vi "Get INI Section.vi"(4 "section name":string="desktop", 5 "file content":string="[windows]\nspooler=no\nNetWarn=1\nNetMessage=Yes\nload=c:\\windows\\number9\\hawkeye.exe C:\\MOUSE\\pointer.exe\n\nrun=c:\\DELL\\WINBATCH.EXE\nBeep=yes\nNullPort=None\ndevice=\nBorderWidth=3\nCursorBlinkRate=530\nDoubleClickSpeed=452\nPrograms=com exe bat pif\nDocuments=\nDeviceNotSelectedTimeout=15\nTransmissionRetryTimeout=45\nKeyboardDelay=2\nKeyboardSpeed=31\nScreenSaveActive=0\nScreenSaveTimeOut=120\n\n[Desktop]\noldwallpaper=dell1.bmp\nPattern=(None)\nTileWallpaper=1\nGridGranularity=0\n\n[Extensions]\ncal=calendar.exe ^.cal\ncrd=cardfile.exe ^.crd\ntrm=terminal.exe ^.trm\ntxt=notepad.exe ^.txt\nini=notepad.exe ^.ini\npcx=pbrush.exe ^.pcx\nbmp=pbrush.exe ^.bmp\nwri=write.exe ^.wri\nrec=recorder.exe ^.rec\nhlp=winhelp.exe ^.hlp\n\n[intl]\nsLanguage=enu\nsCountry=United States\niCountry=1\niDate=0\niTime=0\niTLZero=0\niCurrency=0\niCurrDigits=2\niNegCurr=0\niLzero=1\niDigits=2\niMeasure=1\ns1159=AM\ns2359=PM\nsCurrency=$\nsThousand=,\nsDecimal=.\nsDate=/\nsTime=:\nsList=,\nsShortDate=M/d/yy\nsLongDate=dddd, MMMM dd, yyyy\n\n[ports]\n; A line with [filename].PRN followed by an equal sign causes\n; [filename] to appear in the Control Panel's Printer Configuration dialog\n; box. A printer connected to [filename] directs its output into this file.\nLPT1:=\nLPT2:=\nLPT3:=\nCOM1:=9600,n,8,1,x\nCOM2:=9600,n,8,1,x\nCOM3:=9600,n,8,1,x\nCOM4:=9600,n,8,1,x\nEPT:=\nFILE:=\nLPT1.DOS=\nLPT2.DOS=\n\n[FontSubstitutes]\nHelv=MS Sans Serif\nTms Rmn=MS Serif\nTimes=Times New Roman\nHelvetica=Arial\n\n[TrueType]\n\n[Sounds]\nRingOut=ringout.wav,Chat Outgoing Ring\nRingIn=ringin.wav,Chat Incoming Ring\nSystemDefault=ding.wav, Default Beep\nSystemExclamation=chord.wav, Exclamation\nSystemStart=tada.wav, Windows Start\nSystemExit=chimes.wav, Windows Exit\nSystemHand=chord.wav, Critical Stop\nSystemQuestion=chord.wav, Question\nSystemAsterisk=chord.wav, Asterisk\n\n[mci extensions]\nwav=waveaudio\nmid=sequencer\nrmi=sequencer\n\n[Compatibility]\nTURBOTAX=0x00080000\nW4GLR=0x4000\nW4GL=0x4000\nNETSET2=0x0100\nGUIDE=0x1000\nEXCEL=0x1000\nAPORIA=0x0100\nED=0x00010000\nPLUS=0x1000\nPR2=0x2000\nCHARISMA=0x2000\nWINSIM=0x2000\nDRAW=0x2000\nPLANNER=0x2000\nDESIGNER=0x2000\nPM4=0x2000\nMILESV3=0x1000\n_BNOTES=0x24000\nMCOURIER=0x0800\nVISION=0x0040\nPACKRAT=0x0800\nWIN2WRS=0x1210\nVB=0x0200\nTME=0x0100\nJW=0x42080\nCP=0x0040\nPIXIE=0x0040\nREM=0x8022\nAMIPRO=0x0010\nCCMAIL=0x0008\nWPWINFIL=0x0006\nNOTSHELL=0x0001\n\n[Microsoft Word 2.0]\nHPDSKJET=+1\n\n[wt4gpi8s56bz]\nArial (TrueType)=ARIAL.FOT\nArial Bold (TrueType)=ARIALBD.FOT\nArial Bold Italic (TrueType)=ARIALBI.FOT\nArial Italic (TrueType)=ARIALI.FOT\nCourier New (TrueType)=COUR.FOT\nCourier New Bold (TrueType)=COURBD.FOT\nCourier New Bold Italic (TrueType)=COURBI.FOT\nCourier New Italic (TrueType)=COURI.FOT\nTimes New Roman (TrueType)=TIMES.FOT\nTimes New Roman Bold (TrueType)=TIMESBD.FOT\nTimes New Roman Bold Italic (TrueType)=TIMESBI.FOT\nTimes New Roman Italic (TrueType)=TIMESI.FOT\nWingDings (TrueType)=WINGDING.FOT\nMS Sans Serif 8,10,12,14,18,24 (VGA res)=SSERIFE.fon\nCourier 10,12,15 (VGA res)=COURE.fon\nMS Serif 8,10,12,14,18,24 (VGA res)=SERIFE.fon\nSymbol 8,10,12,14,18,24 (VGA res)=SYMBOLE.fon\nRoman (Plotter)=ROMAN.FON\nScript (Plotter)=SCRIPT.FON\nModern (Plotter)=MODERN.FON\nSmall Fonts (VGA res)=SMALLE.fon\nHelv 8,10,12,14,18,24 (1280 res)=HELVF.FON\nTms Rmn 8,10,12,14,18,24 (1280 res)=TMSRF.FON\nCourier 10,12,15 (1280 res)=COURF.FON\nSymbol (TrueType)=SYMBOL.FOT\n\n[embedding]\nSoundRec=Sound,Sound,SoundRec.exe,picture\nPackage=Package,Package,packager.exe,picture\nPBrush=Paintbrush Picture,Paintbrush Picture,pbrush.exe,picture\n\n[winsetup]\nsource_disk_path=a:\\\n") -> (0 "after section":string, 1 "section":string[](array[string]), 2 "before section":string)   [LabVIEW 2020, in "NI_FTP.lvlib"]
uses:
  <vilib>/FTP/NI_FTP.lvlib
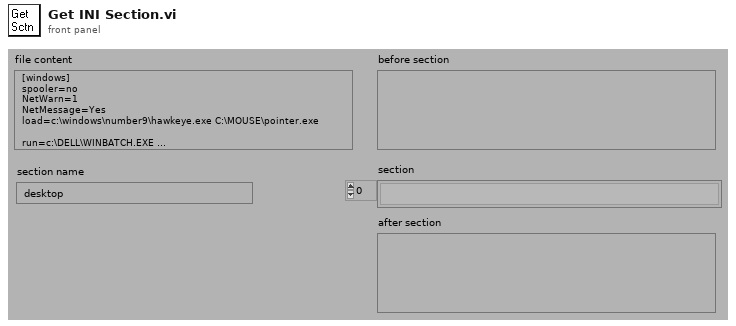
[diagram p1: front panel]
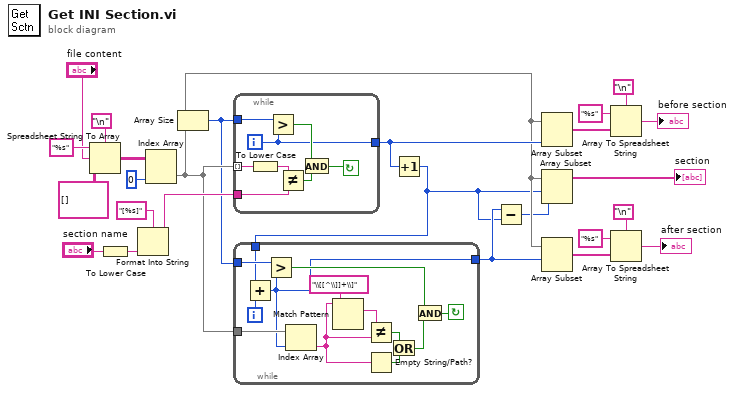
[diagram p0: block diagram]
diagram:
  n1 = Spreadsheet String To Array(delimiter (Tab)="\n", format string="%s", spreadsheet string="file content", array type (2D Dbl)=string[][] []) -> (array=w22:string[][])
  n2 = To Lower Case(string="section name") -> (all lower case string=w18:string)
  n3 = Format Into String(format string="[%s]", w18) -> (resulting string=w16:string)  [unwired: 2 in, 1 out]
  n4 = Index Array(array=w22, index (col)=0) -> (element=w6:string[])  [unwired: 1 in]
  n5 = Array Size(array=w6) -> (size(s)=w3:i32)
  n6 = while {
    tunnel: [w26] -> w15
    tunnel: w3 -> [w30]
    tunnel: w16 -> [w32]
    tunnel: w6 -> [w33] mode=indexing
    i -> [w26]
    stop <- w27 continue-if-true
    n7 = To Lower Case(string=w33) -> (all lower case string=w31:string)
    n8 = Greater?(x=w30, y=w26) -> (0:w29:bool)
    n9 = Not Equal?(x=w31, y=w32) -> (x != y?=w28:bool)
    n10 = And(x=w29, y=w28) -> (x .and. y?=w27:bool)
  }
  n11 = Increment(x=w15) -> (x+1=w1:i32)
  n12 = while {
    tunnel: [w34] -> w2
    tunnel: w1 -> [w36]
    tunnel: w3 -> [w44]
    tunnel: w6 -> [w43]
    i -> [w45]
    stop <- w40 continue-if-true
    n13 = Add(x=w36, y=w45) -> (x+y=w34:i32)
    n14 = Greater?(x=w44, y=w34) -> (0:w41:bool)
    n15 = Index Array(array=w43, index=w34) -> (element=w39:string)
    n16 = Match Pattern(string=w39, regular expression="\\[[^\\]]+\\]") -> (match substring=w42:string)  [unwired: 4 out]
    n17 = Not Equal?(x=w42, y=w39) -> (x != y?=w37:bool)
    n18 = Empty String/Path?(string/path=w39) -> (empty?=w35:bool)
    n19 = Or(x=w37, y=w35) -> (x .or. y?=w38:bool)
    n20 = And(x=w41, y=w38) -> (x .and. y?=w40:bool)
  }
  n21 = Subtract(x=w2, y=w1) -> (x-y=w4:i32)
  n22 = Array Subset(array=w6, length=w15) -> (w14:string[])  [unwired: 1 in]
  n23 = Array Subset(array=w6, index=w1, length=w4) -> (→"section":string[])
  n24 = Array Subset(array=w6, index=w2) -> (w8:string[])  [unwired: 1 in]
  n25 = Array To Spreadsheet String(delimiter (Tab)="\n", array=w14, 3:"%s" ("format string")) -> (spreadsheet string=→"before section":string)
  n26 = Array To Spreadsheet String(delimiter (Tab)="\n", array=w8, 3:"%s" ("format string")) -> (spreadsheet string=→"after section":string)
